vi "Convert_calc_app-spec_preview_graphs.vi"(7 "data from unit":u8, 8 "Labels in":string[](array[string]), 9 "Values in mV in":dbl[](array[numeric]), 10 "Conversion settings":T1={"Fxn array names 2"=[[0, 0, 1], [0, 0, 0], [0, 0, 0], [0, 2, 3], [0, 0, 0], [0, 0, 0], [0, 0, 0], [0, 0, 0], [0, 0, 0], [0, 0, 0], [0, 0, 0], [0, 0, 0]], "Unit conf cat. 2"=["10,11,12", "13,14", "15"]} {"Fxn array names 2" items=["c", "O2 %", "CO ppm", "new", "aa"]}, 11 "Formulas definitions":string[][](table)=[["c", "1E6*volt"], ["O2 %", "exp(-20.0*volt)"], ["CO ppm", "5*volt"], ["new", "volt"]]) -> (1 "Labels out":string[](array[string]), 2 "Values converted out":dbl[](array[numeric]) format="%#_6e")   [LabVIEW 2013]
uses:
  Converter_app_spec_set.ctl
  <vilib>/gmath/NI_Gmath.lvlib
panel:
  out "eq filled in x":string
  # "Comma separated unit selection (-1 keyword for others)"
  # "A1.0"
  # "A1.1"
  # "A1.2"
  # "A1.3"
  # "A2.0"
  # "A2.1"
  # "A2.2"
  # "A2.3"
  # "A3.0"
  # "A3.1"
  # "A3.2"
  # "A3.3"
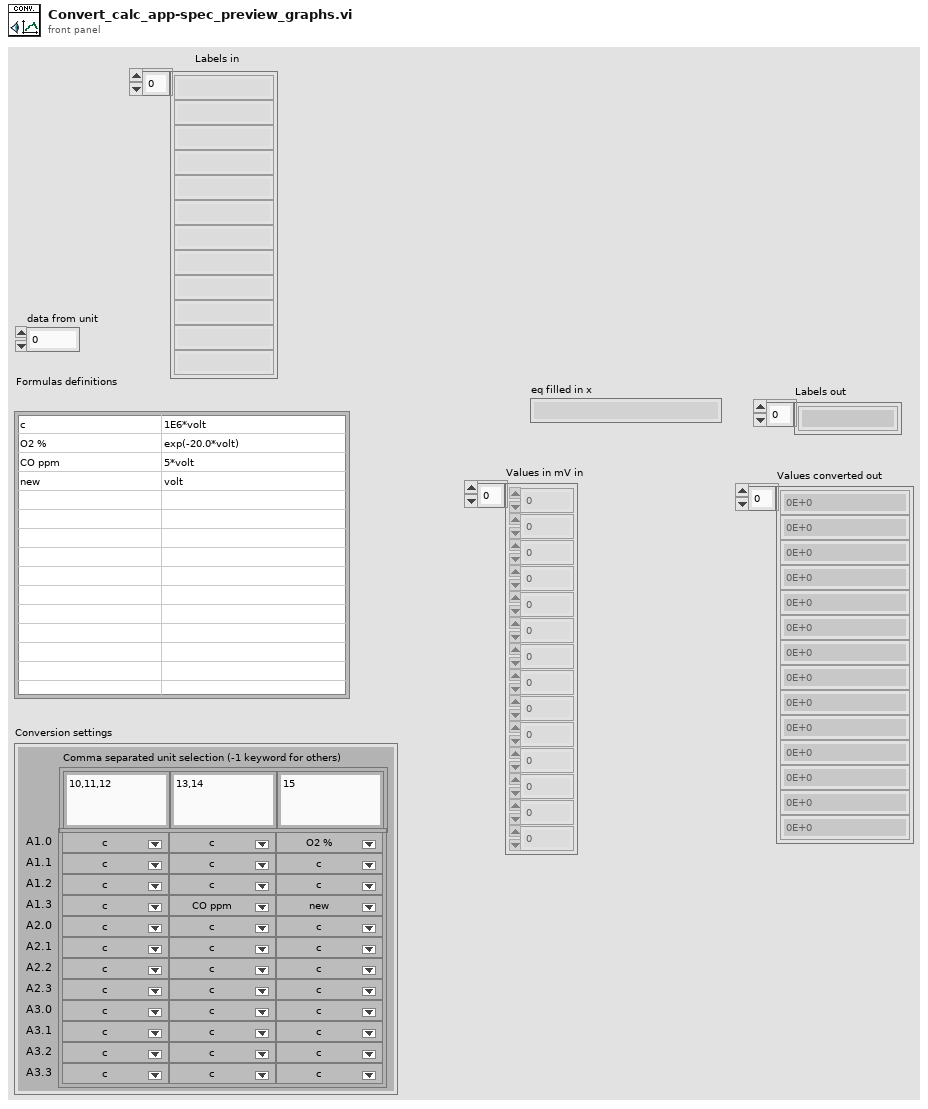
[diagram p1: front panel]
types:
  T1 = typedef "Converter_app_spec_set.ctl" = cluster{"Fxn array names 2":u16[][], "Unit conf cat. 2":string[]}
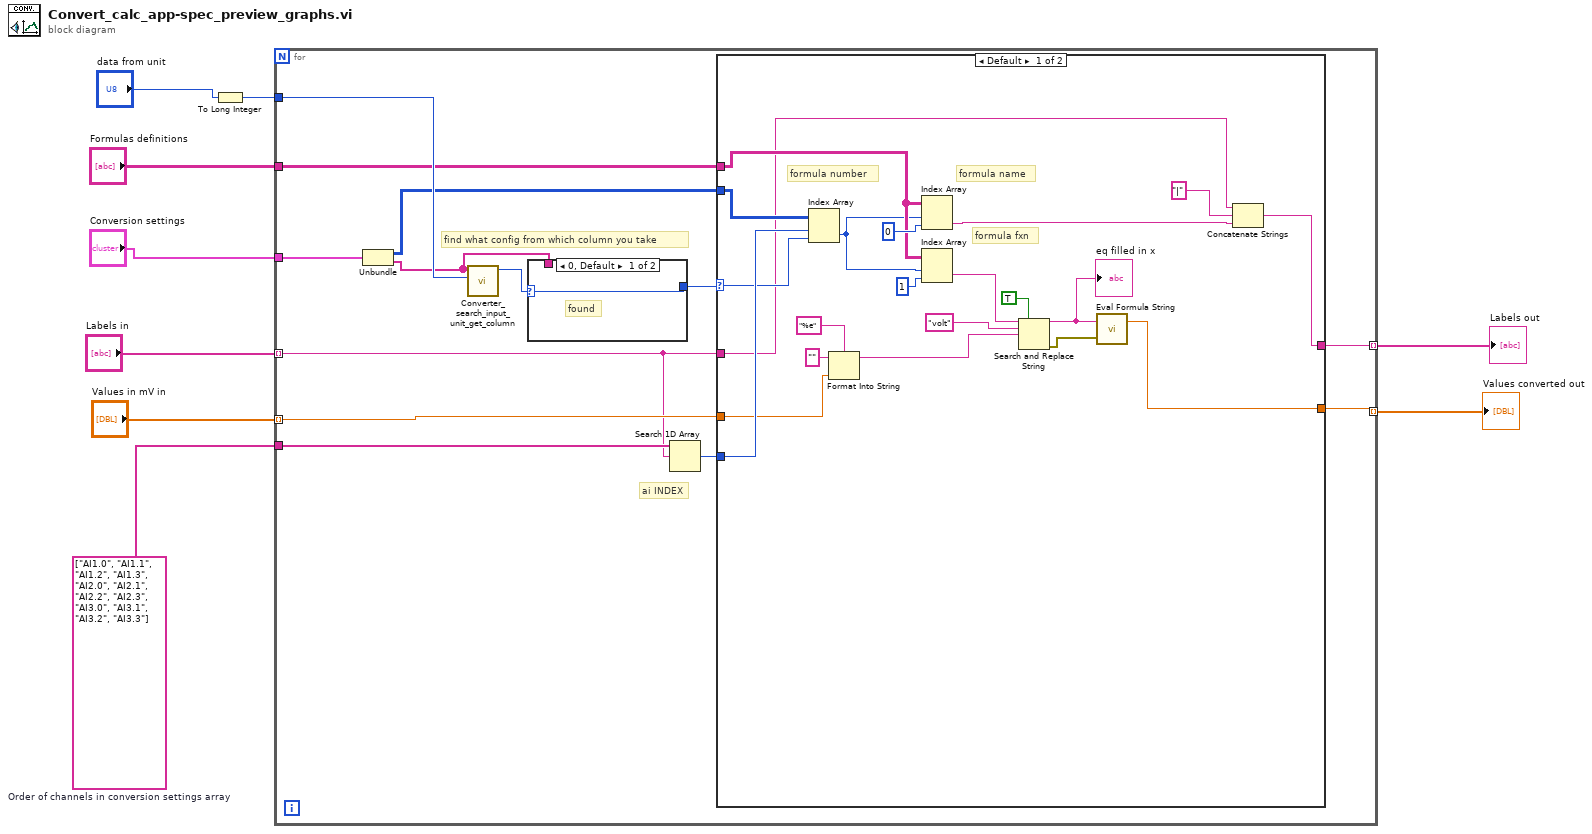
[diagram p0: block diagram]
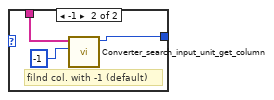
[diagram p3: hidden frame]
diagram:
  w2 = string[] ["AI1.0", "AI1.1", "AI1.2", "AI1.3", "AI2.0", "AI2.1", "AI2.2", "AI2.3", "AI3.0", "AI3.1", "AI3.2", "AI3.3"]  # Order of channels in conversion settings array
  n1 = To Long Integer(number="data from unit") -> (32bit integer=w7:i32)
  n2 = for {
    tunnel: "Conversion settings" -> [w22]
    tunnel: w7 -> [w21]
    tunnel: "Labels in" -> [w13] mode=indexing
    tunnel: "Values in mV in" -> [w17] mode=indexing
    tunnel: [w16] -> w4 mode=indexing
    tunnel: [w15] -> w3 mode=indexing
    tunnel: w2 -> [w14]
    tunnel: "Formulas definitions" -> [w11]
    # "ai INDEX"
    # "find what config from which column you take"
    n3 = Unbundle(w22) -> ("Fxn array names 2"=w10:u16[][], "Unit conf cat. 2"=w19:string[])
    n4 = call "Converter_search_input_unit_get_column.vi"("unit to search for"=w21, "Unit conf cat. in"=w19) -> ("found in column number"=w20:i32)  [unwired: 9 in]
    n5 = case shown="0, Default" w20 {
      selector: w20 -> [w46 _]
      tunnel: [w46 w47] -> w18
      tunnel: w19 -> [_ w49]
      frame 0, Default {
        # "found"
      }
      frame -1 {
        # "filnd col. with -1 (default)"
        n6 = call "Converter_search_input_unit_get_column.vi"("unit to search for"=-1, "Unit conf cat. in"=w49) -> ("found in column number"=w47:i32)  [unwired: 9 in]
      }
    }
    n7 = Search 1D Array(1D array=w14, element=w13) -> (index of element=w12:i32)  [unwired: 1 in]
    n8 = case shown="Default" w18 {
      selector: w18 -> [w41 _]
      tunnel: w13 -> [w25 w44]
      tunnel: w17 -> [w32 w45]
      tunnel: [w28 w45] -> w16
      tunnel: [w26 w44] -> w15
      tunnel: w12 -> [w42 _]
      tunnel: w11 -> [w38 _]
      tunnel: w10 -> [w43 _]
      frame Default {
        # "formula fxn"
        # "formula name"
        # "formula number"
        n9 = Index Array(array=w43, index (row)=w42, index (col)=w41) -> (element=w37:u16)
        n10 = Format Into String(format string="%e", initial string="", w32) -> (resulting string=w33:string)  [unwired: 1 in, 1 out]
        n11 = Index Array(array=w38, index (row)=w37, index (col)=0 ("disabled index (col)")) -> (element=w24:string)
        n12 = Index Array(array=w38, index (row)=w37, index (col)=1 ("disabled index (col)")) -> (element=w34:string)
        n13 = Search and Replace String(replace all?=TRUE ("replace all? (F)"), input string=w34, search string="volt", replace string=w33) -> (result string=w29:string, error out=w27:errorcluster)  [unwired: 4 in, 2 out]
        "eq filled in x" <- w29
        n14 = call <vilib>:"Eval Formula String.vi"("error in (no error)"=w27, "formula"=w29) -> ("y value"=w28:dbl)  [unwired: 1 out]
        n15 = Concatenate Strings(w25, "|" ("string"), w24) -> (w26:string)
      }
      frame -1 {
        # "no settings found for the current unit \nand no default was set (no -1 in selector)"
      }
    }
  }
  "Values converted out" <- w4
  "Labels out" <- w3
